vi "Images.vi"() -> ()   [LabVIEW 2015]
uses:
  TronviewPresentation/TronviewPresentation/Images.ctl
  TronviewPresentation/TronviewPresentation.lvlib
panel:
  in  "initialized array":T1[][](array[typedef])=[[enum."empty.png", enum."empty.png", enum."empty.png", enum."p1_wall_SE.png", enum."p1_wall_SW.png", enum."empty.png", enum."empty.png", enum."empty.png", enum."empty.png", enum."empty.png"], [enum."p1_pos_W.png", enum."p1_wall_EW.png", enum."p1_wall_EW.png", enum."p1_wall_NW.png", enum."p1_wall_NE.png", enum."p1_pos_E.png", enum."empty.png", enum."empty.png", enum."empty.png", enum."empty.png"], [enum."p1_pos_N.png", enum."p2_pos_W.png", enum."p2_wall_EW.png", enum."p2_wall_SW.png", enum."p2_wall_SE.png", enum."p2_pos_E.png", enum."empty.png", enum."empty.png", enum."empty.png", enum."empty.png"], [enum."p1_wall_NS.png", enum."empty.png", enum."empty.png", enum."p2_wall_NE.png", enum."p2_wall_NW.png", enum."p2_pos_N.png", enum."empty.png", enum."empty.png", enum."empty.png", enum."empty.png"], [enum."p1_pos_S.png", enum."empty.png", enum."empty.png", enum."empty.png", enum."empty.png", enum."p2_wall_NS.png", enum."empty.png", enum."empty.png", enum."empty.png", enum."empty.png"], [enum."empty.png", enum."empty.png", enum."empty.png", enum."empty.png", enum."empty.png", enum."p2_pos_S.png", enum."empty.png", enum."empty.png", enum."empty.png", enum."empty.png"], [enum."empty.png", enum."empty.png", enum."empty.png", enum."empty.png", enum."empty.png", enum."empty.png", enum."empty.png", enum."empty.png", enum."empty.png", enum."empty.png"], [enum."empty.png", enum."empty.png", enum."empty.png", enum."empty.png", enum."empty.png", enum."empty.png", enum."empty.png", enum."empty.png", enum."empty.png", enum."empty.png"], [enum."empty.png", enum."empty.png", enum."empty.png", enum."empty.png", enum."empty.png", enum."empty.png", enum."empty.png", enum."empty.png", enum."empty.png", enum."empty.png"], [enum."empty.png", enum."empty.png", enum."empty.png", enum."empty.png", enum."empty.png", enum."empty.png", enum."empty.png", enum."empty.png", enum."empty.png", enum."empty.png"]]
  out "Array 3":picture[][](array[picture])
  out "Array 2":picture[](array[picture])
  out "filenames":string[](array[string])
  in  "path":path
  out "Array":picture[][](array[picture])
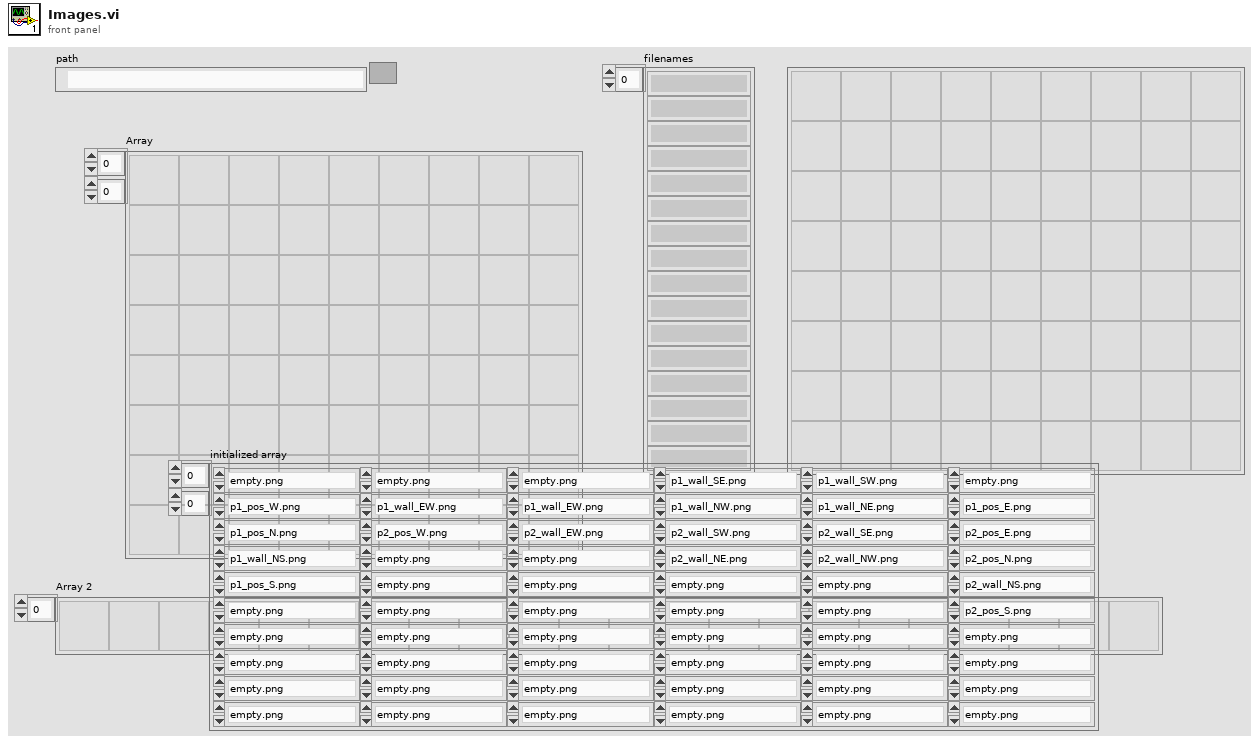
[diagram p1: front panel]
types:
  T1 = typedef "TronviewPresentation.lvlib/Images.ctl" = enum16{"empty.png", "p1_pos_E.png", "p1_pos_N.png", "p1_pos_S.png", "p1_pos_W.png", "p1_wall_EW.png", "p1_wall_NE.png", "p1_wall_NS.png", "p1_wall_NW.png", "p1_wall_SE.png", "p1_wall_SW.png", "p2_pos_E.png", "p2_pos_N.png", "p2_pos_S.png", "p2_pos_W.png", "p2_wall_EW.png", "p2_wall_NE.png", "p2_wall_NS.png", "p2_wall_NW.png", "p2_wall_SE.png", "p2_wall_SW.png"}
  T2 = typedef "imagedata.ctl" = cluster{"image type":i32, "image depth":i32, "image":u8[], "mask":u8[], "colors":u32[], "Rectangle":cluster{"left":i16, "top":i16, "right":i16, "bottom":i16}}
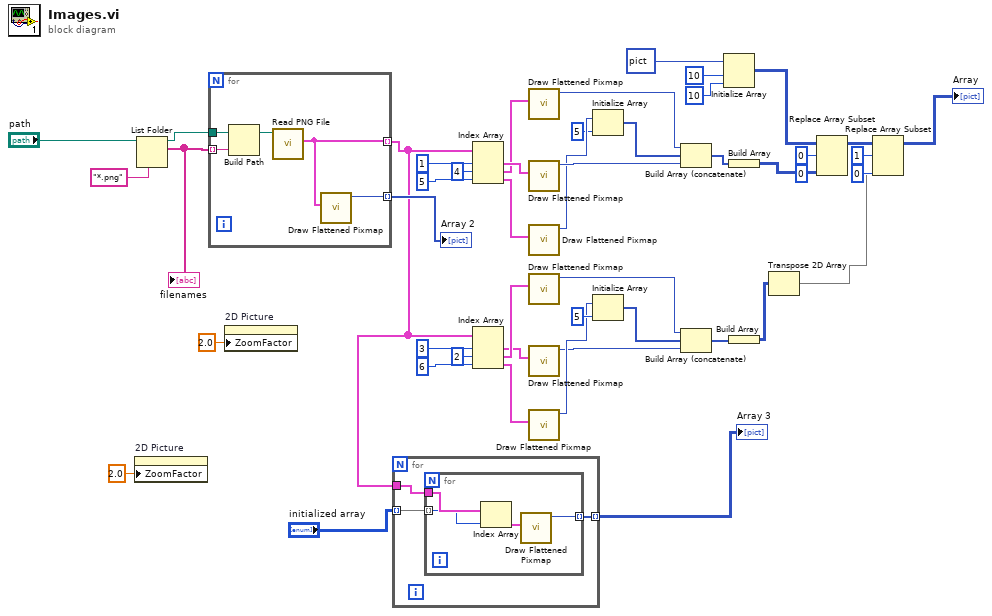
[diagram p0: block diagram]
diagram:
  n1 = property on="2D Picture" class="Pict"("ZoomFactor"=sgl 2.0 ("Zoom Factor")) -> ()  [unwired: 2 in, 2 out]
  n2 = List Folder(path="path", pattern="*.png") -> (path out=w45:path, filenames=w44:string[])  [unwired: 2 in, 2 out]
  "filenames" <- w44
  n3 = for {
    tunnel: w45 -> [w52]
    tunnel: w44 -> [w50] mode=indexing
    tunnel: [w49] -> w4 mode=indexing
    tunnel: [w48] -> w5 mode=indexing
    n4 = Build Path(base path=w52, name or relative path=w50) -> (appended path=w51:path)
    n5 = call <vilib>:"Read PNG File.vi"("path to PNG file"=w51) -> ("image data"=w49:T2)  [unwired: 8 in, 2 out]
    n6 = call <vilib>:"Draw Flattened Pixmap.vi"("image data"=w49) -> ("new picture"=w48:picture)  [unwired: 8 in]
  }
  "Array 2" <- w5
  n7 = property on="2D Picture" class="Pict"("ZoomFactor"=sgl 2.0 ("Zoom Factor")) -> ()  [unwired: 2 in, 2 out]
  n8 = for {
    tunnel: "initialized array" -> [w54] mode=indexing
    tunnel: w4 -> [w55]
    tunnel: [w53] -> w3 mode=indexing
    n9 = for {
      tunnel: w55 -> [w59]
      tunnel: w54 -> [w56] mode=indexing
      tunnel: [w57] -> w53 mode=indexing
      n10 = Index Array(array=w59, index=w56) -> (element=w58:T2)
      n11 = call <vilib>:"Draw Flattened Pixmap.vi"("image data"=w58) -> ("new picture"=w57:picture)  [unwired: 8 in]
    }
  }
  "Array 3" <- w3
  n12 = Index Array(array=w4, index #1=1 ("index"), index #2=4 ("index"), index #3=5 ("index")) -> (element #1=w42:T2, element #2=w36:T2, element #3=w37:T2)
  n13 = Index Array(array=w4, index #1=3 ("index"), index #2=2 ("index"), index #3=6 ("index")) -> (element #1=w23:T2, element #2=w29:T2, element #3=w28:T2)
  n14 = call <vilib>:"Draw Flattened Pixmap.vi"("image data"=w36) -> ("new picture"=w35:picture)  [unwired: 8 in]
  n15 = call <vilib>:"Draw Flattened Pixmap.vi"("image data"=w42) -> ("new picture"=w41:picture)  [unwired: 8 in]
  n16 = call <vilib>:"Draw Flattened Pixmap.vi"("image data"=w37) -> ("new picture"=w40:picture)  [unwired: 8 in]
  n17 = call <vilib>:"Draw Flattened Pixmap.vi"("image data"=w29) -> ("new picture"=w30:picture)  [unwired: 8 in]
  n18 = call <vilib>:"Draw Flattened Pixmap.vi"("image data"=w23) -> ("new picture"=w24:picture)  [unwired: 8 in]
  n19 = call <vilib>:"Draw Flattened Pixmap.vi"("image data"=w28) -> ("new picture"=w25:picture)  [unwired: 8 in]
  n20 = Initialize Array(w40, 5 ("dimension size")) -> (w34:picture[])
  n21 = Initialize Array(w25, 5 ("dimension size")) -> (w31:picture[])
  n22 = Build Array (concatenate)(w35, w34, w41) -> (w21:picture[])
  n23 = Build Array (concatenate)(w30, w31, w24) -> (w20:picture[])
  n24 = Initialize Array(picture data[5B] ("new picture"), 10 ("dimension size"), 10 ("dimension size")) -> (w15:picture[][])
  n25 = Build Array(w21) -> (w13:picture[][])
  n26 = Build Array(w20) -> (w10:picture[][])
  n27 = Transpose 2D Array(2D array=w10) -> (transposed array=w6:picture[][])
  n28 = Replace Array Subset(array=w15, new element=w13, index (row)=0, index (col)=0 ("disabled index (col)")) -> (w11:picture[][])
  n29 = Replace Array Subset(array=w11, new element=w6, index (row)=1, index (col)=0 ("disabled index (col)")) -> (→"Array":picture[][])
